vi "VoltageRead.vi"(8 "error in":errorcluster, 11 "refnum":refnum<file>) -> (0 "error out":errorcluster, 3 "refnum out":refnum<file>)   [LabVIEW 2009]
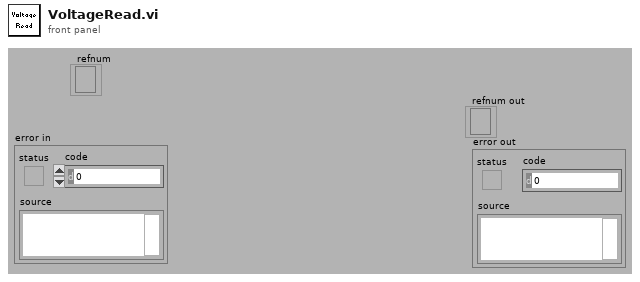
[diagram p1: front panel]
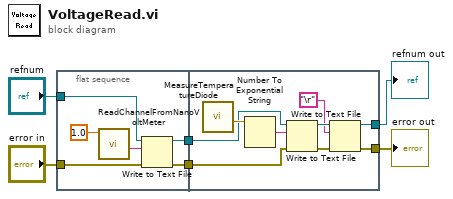
[diagram p0: block diagram]
diagram:
  n1 = flat-sequence {
    tunnel: "refnum" -> [w12]
    tunnel: "error in" -> [w10]
    tunnel: [w8] -> w2
    tunnel: [w7] -> w1
    tunnel: [w16] -> w4
    tunnel: [w15] -> w3
    tunnel: w2 -> [w14]
    tunnel: w1 -> [w13]
    frame #0 {
      n2 = call "ReadChannelFromNanoVoltMeter.vi"("ChannelSelection"=1.0) -> ("String Measurement"=w11:string)  [unwired: 8 in, 2 out]
      n3 = Write to Text File(file (use dialog)=w12, text=w11, error in=w10) -> (refnum out=w7:refnum<file>, error out=w8:errorcluster)  [unwired: 1 in, 1 out]
    }
    frame #1 {
      n4 = call "MeasureTemperatureDiode.vi"() -> ("Celcius"=w18:dbl)  [unwired: 8 in, 3 out]
      n5 = Number To Exponential String(number=w18) -> (E-format string=w21:string)  [unwired: 3 in]
      n6 = Write to Text File(file (use dialog)=w13, text=w21, error in=w14) -> (refnum out=w19:refnum<file>, error out=w20:errorcluster)  [unwired: 1 in, 1 out]
      n7 = Write to Text File(file (use dialog)=w19, text="\r", error in=w20) -> (refnum out=w16:refnum<file>, error out=w15:errorcluster)  [unwired: 1 in, 1 out]
    }
  }
  "refnum out" <- w4
  "error out" <- w3
